vi "API - Add Rx Channels.vi"(8 "error in (no error)":errorcluster, 10 "Channel Data":T1 {"Destination Ref" format="%.0x"}, 11 "Packet Ref In":T2=18446744073709551615 format="%.0x") -> (0 "error out":errorcluster, 2 "New Channel Ref":T2=18446744073709551615 format="%.0x", 3 "Packet Ref Out":T2=18446744073709551615 format="%.0x")   [LabVIEW 2016, in "UDP-Custom-Device System Explorer.lvlib"]
uses:
  UDP-Custom-Device System Explorer.lvlib
  <vilib>/NI Veristand/Custom Device API/Custom Device Item Ref.ctl
  TypeDef - Channel Data.ctl
  Shared/DataTypes.ctl
  <vilib>/NI Veristand/Custom Device API/Custom Device Channel.ctl
  <vilib>/NI Veristand/Custom Device API/Custom Device Channel Type.ctl
  Shared/Constants.vi
  <vilib>/NI VeriStand/Custom Device API/Custom Device API.lvlib
  Shared/UDP-Custom-Device Shared.lvlib
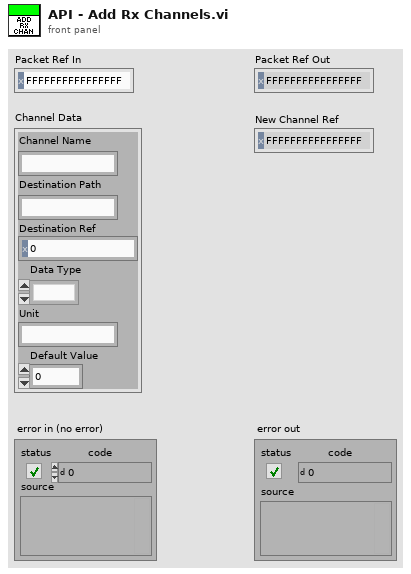
[diagram p1: front panel]
types:
  T1 = typedef "UDP-Custom-Device System Explorer.lvlib/TypeDef - Channel Data.ctl" = cluster{"Channel Name":string, "Destination Path":string, "Destination Ref":T2, "Data Type":T3, "Unit":string, "Default Value":dbl}
  T2 = typedef "Custom Device API.lvlib/Custom Device Item Ref.ctl" = u64
  T3 = typedef "UDP-Custom-Device Shared.lvlib/DataTypes.ctl" = enum16{""}
  T4 = typedef "Custom Device API.lvlib/Custom Device Channel.ctl" = cluster{"Type":T5, "Units":string, "Default Value":dbl, "Faultable":bool, "Scalable":bool}
  T5 = typedef "Custom Device API.lvlib/Custom Device Channel Type.ctl" = enum16{"Input", "Output"}
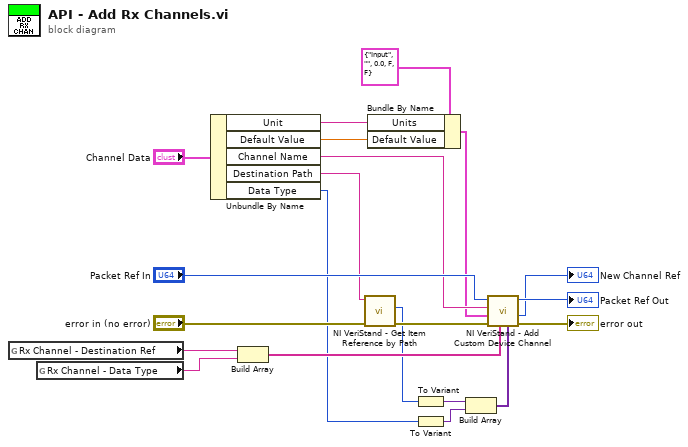
[diagram p0: block diagram]
diagram:
  n1 = global read "Constants.vi" "Rx Channel - Destination Ref"() -> (w14:string)
  n2 = global read "Constants.vi" "Rx Channel - Data Type"() -> (w13:string)
  n3 = Unbundle By Name("Channel Data") -> ("Unit"=w9:string, "Default Value"=w8:dbl, "Channel Name"=w7:string, "Destination Path"=w2:string, "Data Type"=w1:T3)
  n4 = Build Array(w14, w13) -> (w12:string[])
  n5 = call <vilib>:"NI VeriStand - Get Item Reference by Path.vi"("error in (no error)"="error in (no error)", "Item Path in"=w2) -> ("error out"=w4:errorcluster, "Item Ref"=w3:T2)  [unwired: 6 in, 2 out]
  n6 = Bundle By Name(cluster=T4 {"Type"=enum."Input", "Units"="", "Default Value"=0.0, "Faultable"=FALSE, "Scalable"=FALSE} ("Channel"), "Units"=w9, "Default Value"=w8) -> (w6:T4)
  n7 = To Variant(anything=w3) -> (Variant=w17:variant)
  n8 = To Variant(anything=w1) -> (Variant=w16:variant)
  n9 = Build Array(w17, w16) -> (w15:variant[])
  n10 = call <vilib>:"NI VeriStand - Add Custom Device Channel.vi"("Property Values"=w15, "Property names"=w12, "error in (no error)"=w4, "Channel"=w6, "Channel Name"=w7, "Parent Ref in"="Packet Ref In") -> ("error out"=→"error out":errorcluster, "Channel Ref"=→"New Channel Ref":T2, "Parent Ref out"=→"Packet Ref Out":T2)  [unwired: 2 in, 1 out]
